vi "FPGA_convert_U16-to-memadr.vi"(9 "Numeric":u16) -> (1 "mem adr":u8)   [LabVIEW 2010]
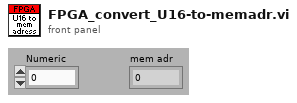
[diagram p1: front panel]
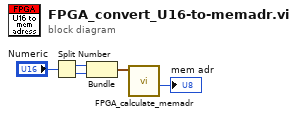
[diagram p0: block diagram]
diagram:
  n1 = Split Number(x="Numeric") -> (hi(x)=w3:u8, lo(x)=w4:u8)
  n2 = Bundle(w3, w4) -> (w1:cluster{u8, u8})  [unwired: 1 out]
  n3 = call "FPGA_calculate_memadr.vi"("Cluster"=w1) -> ("mem adr"=→"mem adr":u8)  [unwired: 10 out]
